vi "Tesla Tester GUI_Main.vi"() -> ()   [LabVIEW 2013, in "Tesla Tester GUI.lvlib"]
uses:
  Tesla Tester GUI.lvlib
  Tesla Tester GUI_Actor/Tesla Tester GUI.lvclass
  <vilib>/ActorFramework/Message Queue/Message Queue.lvclass/Message Queue.ctl
  <vilib>/ActorFramework/Message Enqueuer/Message Enqueuer.lvclass/Message Enqueuer.ctl
  <vilib>/ActorFramework/Message Enqueuer/Enqueue.vi
  <vilib>/ActorFramework/Message Priority Queue/Priority Enqueue.vi
  <vilib>/ActorFramework/Stop Msg/Stop Msg.lvclass
  <vilib>/ActorFramework/Actor/Actor.lvclass
  <vilib>/ActorFramework/Message Queue/Message Queue.lvclass
  Messages/StartMeasurement_Msg/StartMeasurement_Msg.lvclass
panel:
  in  "Run tests":bool
  in  "List of tests":i32(listbox)
  in  "Quit":bool
  in  "Start":bool
  # "Use standard windows/mac stuff here.  Hold 'control' button to select more than one test to run.\nAssuming touch screen, hence large buttons."
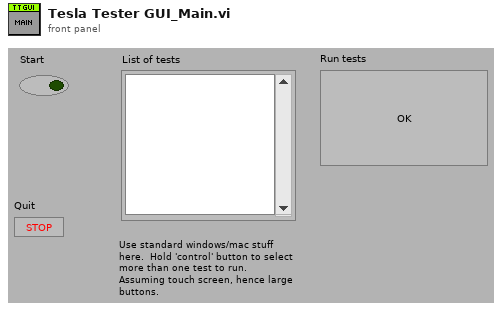
[diagram p1: front panel]
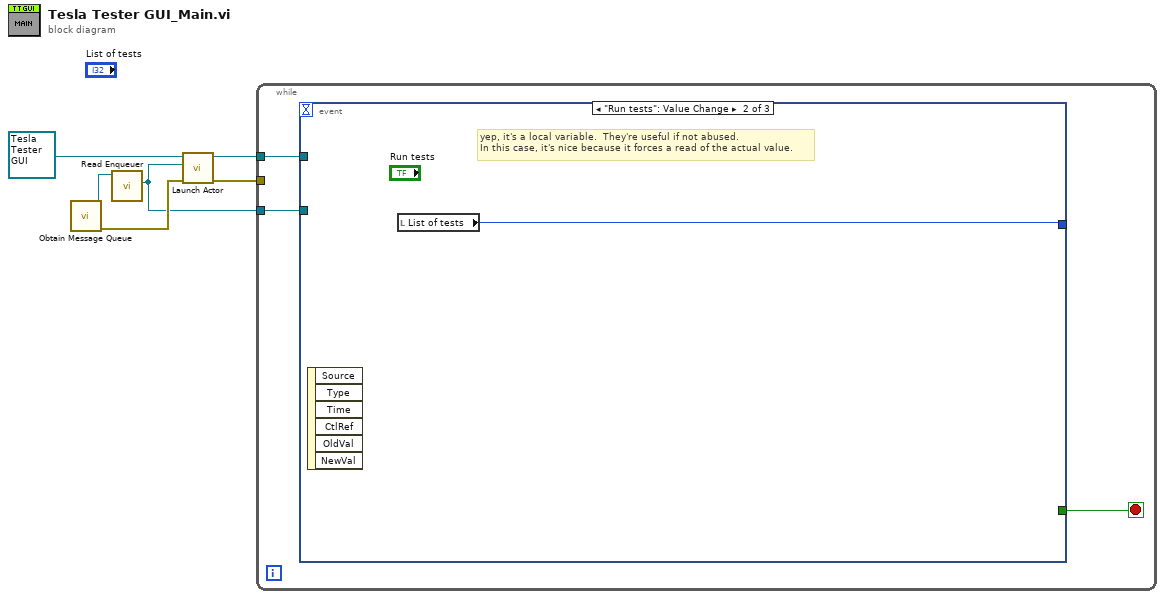
[diagram p0: block diagram]
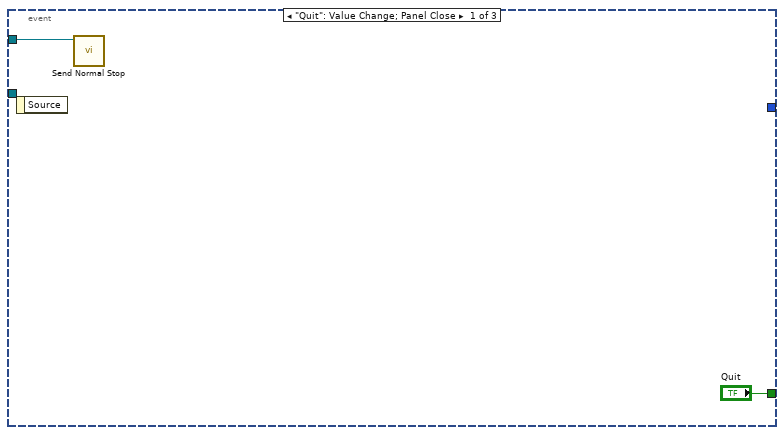
[diagram p2: hidden frame]
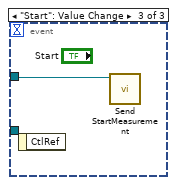
[diagram p3: hidden frame]
diagram:
  n1 = call <vilib>:"Obtain Message Queue.vi"() -> ("error out"=w2:errorcluster, "Message Queue"=w5:refnum<class "Message Queue.lvclass">)  [unwired: 10 in]
  n2 = call <vilib>:"Read Enqueuer.vi"("Message Queue"=w5) -> ("Message Enqueuer"=w1:refnum<class "Message Enqueuer.lvclass">)  [unwired: 10 in]
  n3 = call <vilib>:"Launch Actor.vi"("error in (no error)"=w2, "Actor-to-Caller Enqueuer"=w1, "Actor"=refnum<class "Tesla Tester GUI.lvclass"> refnum ("Actor1_GUI_4.0.0.lvlib:Actor1_GUI")) -> ("error out"=w3:errorcluster, "Caller-To-Actor Enqueuer"=w4:refnum<class "Message Enqueuer.lvclass">)  [unwired: 7 in]
  n4 = while {
    tunnel: w4 -> [w8]
    tunnel: w3 -> [_]
    tunnel: w1 -> [w7]
    stop <- w9 stop-if-true
    n5 = event shown="[1] \"Run tests\": Value Change" {
      selector: _ -> [_ _ _]
      dyn-events: _ -> [_ _ _]
      timeout: _ -> [_ _ _]
      tunnel: ["Quit" _ _] -> w9
      tunnel: w8 -> [w10 _ w13]
      tunnel: w7 -> [_ _ _]
      tunnel: [_ w12 _] -> _
      event "Quit": Value Change; Panel Close {
        n6 = event-data() -> ()  [unwired: 1 in, 1 out]
        n7 = call <vilib>:"Send Normal Stop.vi"("Message Enqueuer"=w10) -> ()  [unwired: 10 in, 1 out]
      }
      event "Run tests": Value Change {
        # "yep, it's a local variable.  They're useful if not abused.\nIn this case, it's nice because it forces a read of the actual value."
        n8 = event-data() -> ()  [unwired: 1 in, 6 out]
        n9 = local read "List of tests"() -> (w12:i32)
      }
      event "Start": Value Change {
        n10 = event-data() -> ()  [unwired: 1 in, 1 out]
        n11 = call "Send StartMeasurement.vi"("Message Enqueuer"=w13) -> ()  [unwired: 10 in, 1 out]
      }
    }
  }
